vi "filter engines by alias.vi"(7 "engine aliases (empty = ALL)":string[](array[string]), 8 "error in (no error)":errorcluster, 11 "target engines":T1[](array[typedef])) -> (0 "error out":errorcluster, 3 "filtered engines":T1[](array[typedef]))   [LabVIEW 2014, in "PL_Target Runtime.lvclass"]
uses:
  PL_Target Runtime.lvclass
  platypus configuration/engines cluster.ctl
  <vilib>/NI/Module Execution Interface/Engine Configuration/engine configuration.lvclass
  <vilib>/NI/Tag Bus Module Framework/module configuration/TBM module configuration.lvclass
  <vilib>/NI/Configuration Framework/serializable configuration/NISE_CEF_serializable configuration.lvclass
  platypus configuration/PLConfigurationSerializer.lvlib
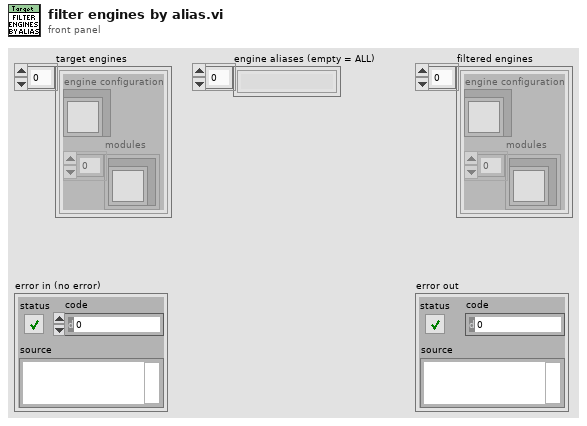
[diagram p1: front panel]
types:
  T1 = typedef "PLConfigurationSerializer.lvlib/engines cluster.ctl" = cluster{"engine configuration":refnum<class "engine configuration.lvclass">, "modules":refnum<class "TBM module configuration.lvclass">[]}
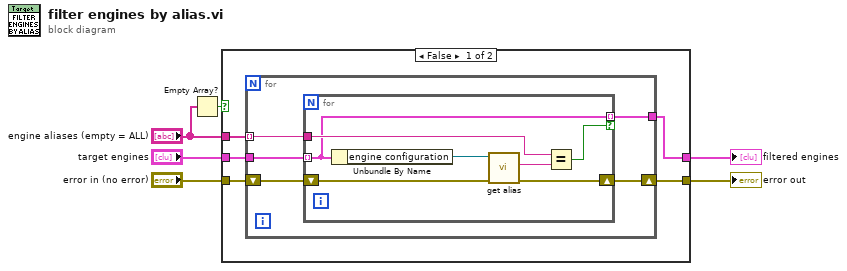
[diagram p0: block diagram]
diagram:
  n1 = Empty Array?(array="engine aliases (empty = ALL)") -> (empty?=w2:bool)
  n2 = case shown="False" w2 {
    tunnel: "engine aliases (empty = ALL)" -> [w11 _]
    tunnel: [w10 w24] -> w6
    tunnel: "error in (no error)" -> [w9 w24]
    tunnel: "target engines" -> [w8 w25]
    tunnel: [w7 w25] -> w1
    frame False {
      n3 = for {
        tunnel: w8 -> [w16]
        tunnel: w11 -> [w13] mode=indexing
        shift-right: [w14] -> w10
        shift-left: w9 -> [w15]
        tunnel: [w12] -> w7
        n4 = for {
          tunnel: w16 -> [w18] mode=indexing
          shift-right: [w21] -> w14
          shift-left: w15 -> [w22]
          tunnel: w13 -> [w19]
          tunnel: [w18] -> w12 mode=indexing if=w17
          n5 = Unbundle By Name(w18) -> ("engine configuration"=w23:refnum<class "engine configuration.lvclass">)
          n6 = call <vilib>:"get alias.vi"("error in"=w22, "configuration in"=w23) -> ("error out"=w21:errorcluster, "alias"=w20:string)  [unwired: 7 in, 1 out]
          n7 = Equal?(x=w19, y=w20) -> (x = y?=w17:bool)
        }
      }
    }
    frame True {
    }
  }
  "filtered engines" <- w1
  "error out" <- w6
